vi "WLAN - TV - RW - UTIL - TestVectors_11A.vi"(0 "TV_IQComposite_11A":T2={"Standard"=0, "Generation Parameters"=[], "OFDM Advanced Controls"={"OFDM Auto Compute Acquisition Length Enabled"=0, "OFDM Maximum Symbols Used"=0, "OFDM Time Tracking Enabled"=0, "OFDM Channel Tracking Enabled"=0, "OFDM Amplitude Tracking Enabled"=1, "OFDM CFO Estimation Method"=0, "OFDM Phase Tracking Method"=0, "OFDM Header Detection Enabled"=0, "OFDM MAC FCS Check Enabled"=0, "#Avg"=0, "#Iterations"=10}, "Measurement  Enabled ?"=FALSE, "#Packets"=0} {"OFDM Advanced Controls"."OFDM Phase Tracking Method" items=["Standard", "Instantaneous", "None", "Standard with Cubic Spline Fit"]; "OFDM Advanced Controls"."OFDM CFO Estimation Method" items=["Preamble Only", "Preamble and Data"]; "OFDM Advanced Controls"."OFDM Channel Tracking Enabled" items=["False", "True"]; "OFDM Advanced Controls"."OFDM Amplitude Tracking Enabled" items=["False", "True"]; "OFDM Advanced Controls"."OFDM Time Tracking Enabled" items=["True"=1, "False"=0]; "OFDM Advanced Controls"."OFDM Auto Compute Acquisition Length Enabled" items=["False", "True"]; "OFDM Advanced Controls"."OFDM MAC FCS Check Enabled" items=["False", "True"]; "OFDM Advanced Controls"."OFDM Header Detection Enabled" items=["False", "True"]; "Generation Parameters"."Payload Control"."OFDM Data Rate (Mbps)" items=["6", "9", "12", "18", "24", "36", "48", "54"]; "Generation Parameters"."Center Frequency(Hz)" format="%#_6p"; "Standard" items=["80211A/G/J/P OFDM", "80211B/G DSSS", "80211G DSSSOFDM", "80211N MIMOOFDM", "80211AC MIMOOFDM"]}, 1 "11a_Meas_Config":path, 3 "TV_802_11a":path, 9 "TV Paramaters":T1) -> ()   [LabVIEW 2011]
uses:
  Includes/WLAN - TV - RW - INC - TV_IQComposite_11A.ctl
  Includes/WLAN - TV - RW - INC - TV_OFDM Demod.ctl
  Includes/WLAN - TV - RW - INC - TV_Parameters.ctl
  Includes/WLAN - TV - RW - INC - Tx_Meas_Settings_OFDM_String.ctl
  <vilib>/Utility/file.llb/Write To Spreadsheet File (string).vi
panel:
  in  "Measurement Type 802.11G":enum32{"Tx Measurement", "Tx Measurement 2"}(tab)
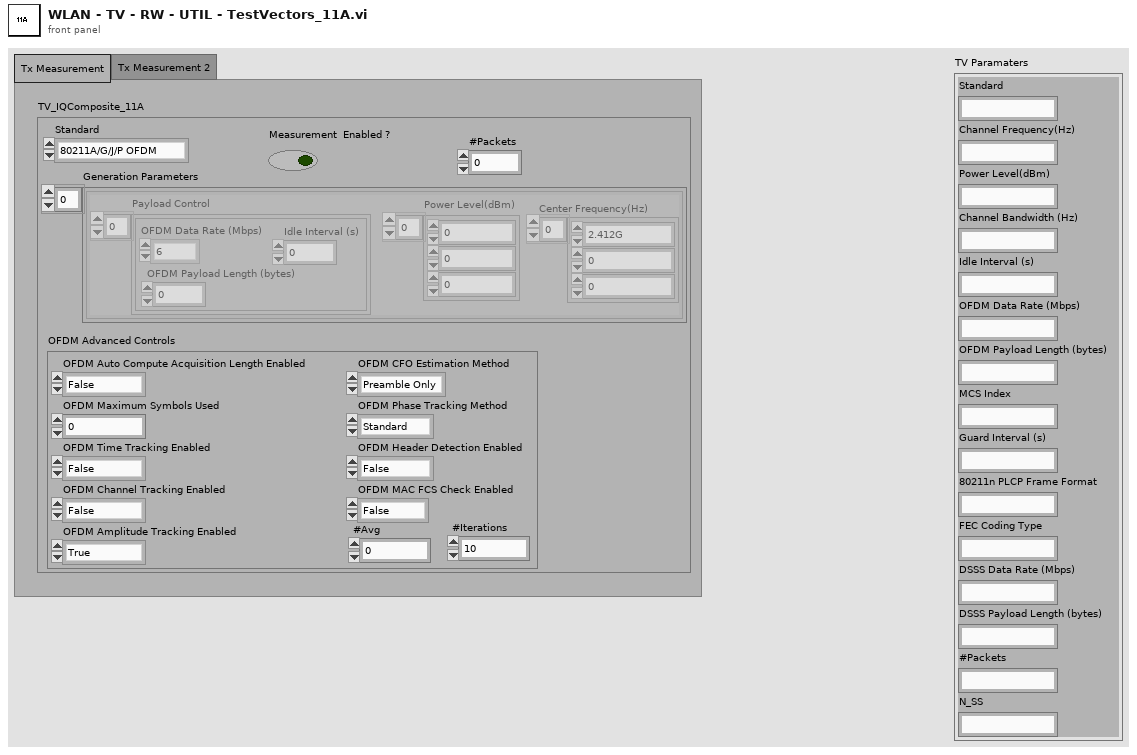
[diagram p1: front panel]
types:
  T1 = typedef "WLAN - TV - RW - INC - TV_Parameters.ctl" = cluster{"Standard ":string, "Channel Frequency(Hz)":string, "Power Level(dBm)":string, "Channel Bandwidth (Hz)":string, "Idle Interval (s)":string, "OFDM Data Rate (Mbps)":string, "OFDM Payload Length (bytes)":string, "MCS Index":string, "Guard Interval (s)":string, "80211n PLCP Frame Format":string, "FEC Coding Type":string, "DSSS Data Rate (Mbps)":string, "DSSS Payload Length (bytes)":string, "#Packets":string, "N_SS":string}
  T2 = typedef "WLAN - TV - RW - INC - TV_IQComposite_11A.ctl" = cluster{"Standard":i32, "Generation Parameters":cluster{"Power Level(dBm)":dbl[], "Center Frequency(Hz)":dbl[], "Payload Control":cluster{"OFDM Data Rate (Mbps)":i32, "OFDM Payload Length (bytes)":i32, "Idle Interval (s)":dbl}[]}[], "OFDM Advanced Controls":T3, "Measurement  Enabled ?":bool, "#Packets":i32}
  T3 = typedef "WLAN - TV - RW - INC - TV_OFDM Demod.ctl" = cluster{"OFDM Auto Compute Acquisition Length Enabled":i32, "OFDM Maximum Symbols Used":i32, "OFDM Time Tracking Enabled":i32, "OFDM Channel Tracking Enabled":i32, "OFDM Amplitude Tracking Enabled":i32, "OFDM CFO Estimation Method":i32, "OFDM Phase Tracking Method":i32, "OFDM Header Detection Enabled":i32, "OFDM MAC FCS Check Enabled":i32, "#Avg":i32, "#Iterations":i32}
  T4 = typedef "WLAN - TV - RW - INC - Tx_Meas_Settings_OFDM_String.ctl" = cluster{"OFDM Auto Compute Acquisition Length Enabled":string, "OFDM Maximum Symbols Used":string, "OFDM Time Tracking Enabled":string, "OFDM Channel Tracking Enabled":string, "OFDM Amplitude Tracking Enabled":string, "OFDM CFO Estimation Method":string, "OFDM Phase Tracking Method":string, "OFDM Header Detection Enabled":string, "OFDM MAC FCS Check Enabled":string, "#Avg":string, "#Iterations":string}
  T5 = cluster{"Power Level(dBm)":dbl[], "Center Frequency(Hz)":dbl[], "Payload Control":cluster{"OFDM Data Rate (Mbps)":i32, "OFDM Payload Length (bytes)":i32, "Idle Interval (s)":dbl}[]}[]
  T6 = cluster{"OFDM Data Rate (Mbps)":i32, "OFDM Payload Length (bytes)":i32, "Idle Interval (s)":dbl}[]
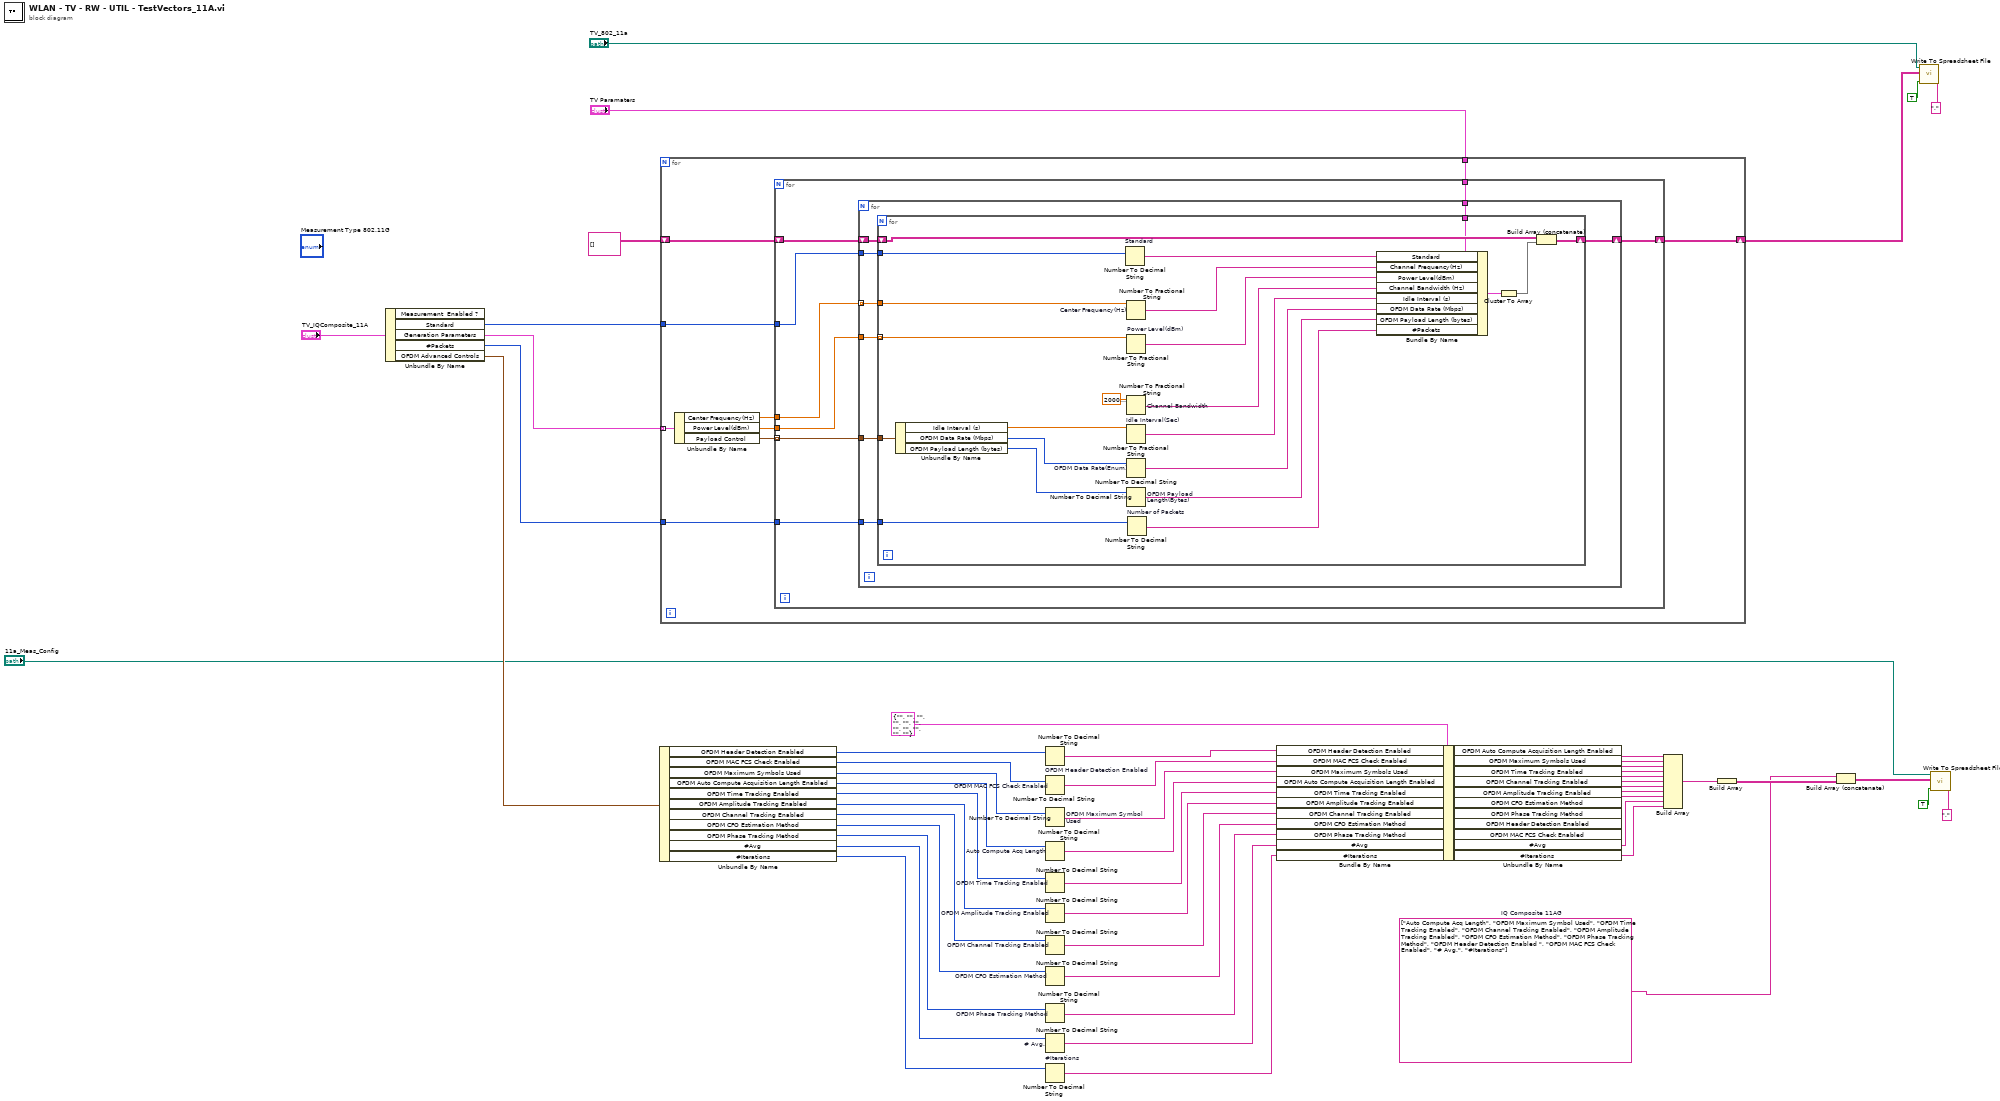
[diagram p0: block diagram]
diagram:
  w2 = string[] ["Auto Compute Acq Length", "OFDM Maximum Symbol Used", "OFDM Time Tracking Enabled", "OFDM Channel Tracking Enabled", "OFDM Amplitude Tracking Enabled", "OFDM CFO Estimation Method", "OFDM Phase Tracking Method", "OFDM Header Detection Enabled ", "OFDM MAC FCS Check Enabled", "# Avg.", "#Iterations"]  # IQ Composite 11AG
  n1 = Unbundle By Name("TV_IQComposite_11A") -> ("Standard"=w53:i32, "Generation Parameters"=w47:T5, "#Packets"=w45:i32, "OFDM Advanced Controls"=w46:T3)  [unwired: 1 out]
  n2 = Unbundle By Name(w46) -> ("OFDM Header Detection Enabled"=w34:i32, "OFDM MAC FCS Check Enabled"=w35:i32, "OFDM Maximum Symbols Used"=w36:i32, "OFDM Auto Compute Acquisition Length Enabled"=w37:i32, "OFDM Time Tracking Enabled"=w38:i32, "OFDM Amplitude Tracking Enabled"=w39:i32, "OFDM Channel Tracking Enabled"=w40:i32, "OFDM CFO Estimation Method"=w41:i32, "OFDM Phase Tracking Method"=w42:i32, "#Avg"=w43:i32, "#Iterations"=w44:i32)
  n3 = for {
    tunnel: w53 -> [w62]
    tunnel: "TV Paramaters" -> [w61]
    tunnel: w47 -> [w60] mode=indexing
    shift-right: [w57] -> w1
    shift-left: string[][] [] ("appended array") -> [w58]
    tunnel: w45 -> [w54]
    n4 = Unbundle By Name(w60) -> ("Center Frequency(Hz)"=w56:dbl[], "Power Level(dBm)"=w55:dbl[], "Payload Control"=w59:T6)
    n5 = for {
      tunnel: w62 -> [w64]
      tunnel: w61 -> [w70]
      tunnel: w59 -> [w65] mode=indexing
      tunnel: w56 -> [w69]
      shift-right: [w67] -> w57
      shift-left: w58 -> [w68]
      tunnel: w55 -> [w66]
      tunnel: w54 -> [w63]
      n6 = for {
        shift-right: [w77] -> w67
        shift-left: w68 -> [w78]
        tunnel: w64 -> [w76]
        tunnel: w70 -> [w75]
        tunnel: w69 -> [w74] mode=indexing
        tunnel: w66 -> [w73]
        tunnel: w65 -> [w72]
        tunnel: w63 -> [w71]
        n7 = for {
          tunnel: w74 -> [w82]
          shift-right: [w100] -> w77
          shift-left: w78 -> [w99]
          tunnel: w76 -> [w98]
          tunnel: w75 -> [w96]
          tunnel: w73 -> [w81] mode=indexing
          tunnel: w72 -> [w88]
          tunnel: w71 -> [w84]
          n8 = Unbundle By Name(w88) -> ("Idle Interval (s)"=w85:dbl, "OFDM Data Rate (Mbps)"=w87:i32, "OFDM Payload Length (bytes)"=w86:i32)
          n9 = Number To Decimal String "Standard"(number=w98) -> (decimal integer string=w89:string)  [unwired: 1 in]
          n10 = Number To Fractional String "Center Frequency(Hz)"(number=w82) -> (F-format string=w90:string)  [unwired: 3 in]
          n11 = Number To Fractional String "Power Level(dBm)"(number=w81) -> (F-format string=w91:string)  [unwired: 3 in]
          n12 = Number To Fractional String "Channel Bandwidth"(number=20000000.0) -> (F-format string=w92:string)  [unwired: 3 in]
          n13 = Number To Fractional String "Idle Interval(Sec)"(number=w85) -> (F-format string=w93:string)  [unwired: 3 in]
          n14 = Number To Decimal String "OFDM Data Rate(Enum)"(number=w87) -> (decimal integer string=w94:string)  [unwired: 1 in]
          n15 = Number To Decimal String "OFDM Payload Length(Bytes)"(number=w86) -> (decimal integer string=w95:string)  [unwired: 1 in]
          n16 = Number To Decimal String "Number of Packets"(number=w84) -> (decimal integer string=w83:string)  [unwired: 1 in]
          n17 = Bundle By Name(cluster=w96, "Standard"=w89, "Channel Frequency(Hz)"=w90, "Power Level(dBm)"=w91, "Channel Bandwidth (Hz)"=w92, "Idle Interval (s)"=w93, "OFDM Data Rate (Mbps)"=w94, "OFDM Payload Length (bytes)"=w95, "#Packets"=w83) -> (w80:T1)
          n18 = Cluster To Array(cluster=w80) -> (array=w79:string[])
          n19 = Build Array (concatenate)(w99, w79) -> (w100:string[][])
        }
      }
    }
  }
  n20 = Number To Decimal String "OFDM Header Detection Enabled"(number=w34) -> (decimal integer string=w32:string)  [unwired: 1 in]
  n21 = Number To Decimal String "OFDM MAC FCS Check Enabled"(number=w35) -> (decimal integer string=w31:string)  [unwired: 1 in]
  n22 = Number To Decimal String "OFDM Maximum Symbol Used"(number=w36) -> (decimal integer string=w30:string)  [unwired: 1 in]
  n23 = Number To Decimal String "Auto Compute Acq Length"(number=w37) -> (decimal integer string=w29:string)  [unwired: 1 in]
  n24 = Number To Decimal String "OFDM Time Tracking Enabled"(number=w38) -> (decimal integer string=w28:string)  [unwired: 1 in]
  n25 = Number To Decimal String "OFDM Amplitude Tracking Enabled"(number=w39) -> (decimal integer string=w27:string)  [unwired: 1 in]
  n26 = Number To Decimal String "OFDM Channel Tracking Enabled"(number=w40) -> (decimal integer string=w22:string)  [unwired: 1 in]
  n27 = Number To Decimal String "OFDM CFO Estimation Method"(number=w41) -> (decimal integer string=w23:string)  [unwired: 1 in]
  n28 = Number To Decimal String "OFDM Phase Tracking Method"(number=w42) -> (decimal integer string=w24:string)  [unwired: 1 in]
  n29 = Number To Decimal String "# Avg."(number=w43) -> (decimal integer string=w25:string)  [unwired: 1 in]
  n30 = Number To Decimal String "#Iterations"(number=w44) -> (decimal integer string=w26:string)  [unwired: 1 in]
  n31 = Bundle By Name(cluster=T4 {"OFDM Auto Compute Acquisition Length Enabled"="", "OFDM Maximum Symbols Used"="", "OFDM Time Tracking Enabled"="", "OFDM Channel Tracking Enabled"="", "OFDM Amplitude Tracking Enabled"="", "OFDM CFO Estimation Method"="", "OFDM Phase Tracking Method"="", "OFDM Header Detection Enabled"="", "OFDM MAC FCS Check Enabled"="", "#Avg"="", "#Iterations"=""} ("OFDM Measurement Settings"), "OFDM Header Detection Enabled"=w32, "OFDM MAC FCS Check Enabled"=w31, "OFDM Maximum Symbols Used"=w30, "OFDM Auto Compute Acquisition Length Enabled"=w29, "OFDM Time Tracking Enabled"=w28, "OFDM Amplitude Tracking Enabled"=w27, "OFDM Channel Tracking Enabled"=w22, "OFDM CFO Estimation Method"=w23, "OFDM Phase Tracking Method"=w24, "#Avg"=w25, "#Iterations"=w26) -> (w19:T4)
  n32 = Unbundle By Name(w19) -> ("OFDM Auto Compute Acquisition Length Enabled"=w18:string, "OFDM Maximum Symbols Used"=w17:string, "OFDM Time Tracking Enabled"=w16:string, "OFDM Channel Tracking Enabled"=w15:string, "OFDM Amplitude Tracking Enabled"=w14:string, "OFDM CFO Estimation Method"=w13:string, "OFDM Phase Tracking Method"=w12:string, "OFDM Header Detection Enabled"=w11:string, "OFDM MAC FCS Check Enabled"=w10:string, "#Avg"=w9:string, "#Iterations"=w8:string)
  n33 = Build Array(w18, w17, w16, w15, w14, w13, w12, w11, w10, w9, w8) -> (w7:string[])
  n34 = Build Array(w7) -> (w5:string[][])
  n35 = Build Array (concatenate)(w2, w5) -> (w6:string[][])
  n36 = call-poly <vilib>:"Write To Spreadsheet File.vi"("delimiter (\\t)"="," ("delimiter (\\t)"), "append to file? (new file:F)"=TRUE, "2D data"=w1, "file path (dialog if empty)"="TV_802_11a") -> ()  [unwired: 4 in, 1 out]
  n37 = call-poly <vilib>:"Write To Spreadsheet File.vi"("delimiter (\\t)"="," ("delimiter (\\t)"), "append to file? (new file:F)"=TRUE, "2D data"=w6, "file path (dialog if empty)"="11a_Meas_Config") -> ()  [unwired: 4 in, 1 out]
